vi "setSettingTCPath.vi"(8 "error in (no error)":errorcluster, 10 "Path":path, 11 "Model in":refnum<class "Model.lvclass">) -> (0 "error out":errorcluster, 3 "Model out":refnum<class "Model.lvclass">)   [LabVIEW 2016, in "Model.lvclass"]
uses:
  Model.lvclass
  ComponentTemplateCore/Settings/SettingsTC/TCSettings.lvclass
  home/andres/ct_cmpuserevents/ComponentTemplateCore/Settings/Settings/Setting.lvclass
  ComponentTemplateCore/Settings/Settings/Setting.lvclass/Setting.ctl
  Model.lvclass/Model.ctl
  ComponentTemplateCore/Settings/Settings/Setting.lvclass
panel:
  in  "TCSettings":refnum<class "TCSettings.lvclass">
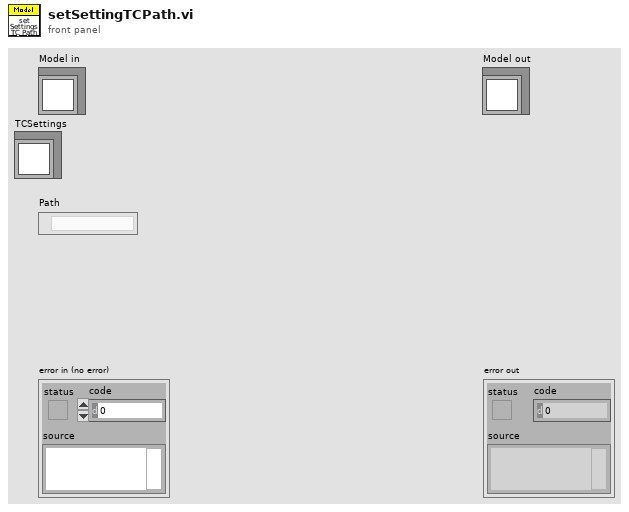
[diagram p1: front panel]
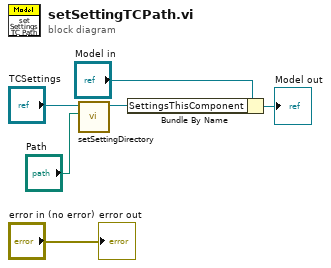
[diagram p0: block diagram]
diagram:
  n1 = call "setSettingDirectory.vi"("SettingDirectory"="Path", "BaseSetting in"="TCSettings") -> ("BaseSetting out"=w1:refnum<class "TCSettings.lvclass">)  [unwired: 9 in]
  n2 = Bundle By Name(cluster="Model in", "SettingsThisComponent"=w1) -> (→"Model out":refnum<class "Model.lvclass">)
  "error out" <- "error in (no error)"
